vi "Module Type.vi"(11 "Event Reporter Module in":refnum<class "Event Reporter Module.lvclass">) -> (2 "Module Type":string)   [LabVIEW 2020, in "Volatus.lvlib" / "Event Reporter Module.lvclass"]
uses:
  Event Reporter Module.lvclass
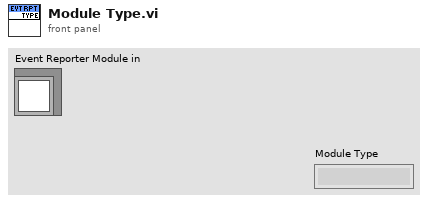
[diagram p1: front panel]
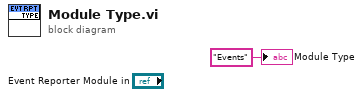
[diagram p0: block diagram]
diagram:
  "Module Type" <- "Events" ("Module Type")
